vi "Get Param.vi"(3 "error in (no error)":errorcluster, 4 "param":dbl, 5 "paramID":i32) -> (0 "error out":errorcluster, 1 "param out":dbl, 2 "function return":i32)   [LabVIEW 2014, in "ThorZStepper.lvlib"]
doc: "long GetParam(const long paramID, double &param);"
uses:
  ThorZStepper.lvlib
  ThorZStepper.dll
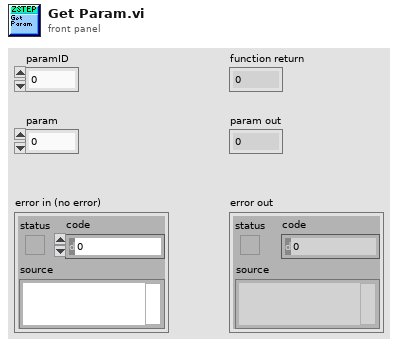
[diagram p1: front panel]
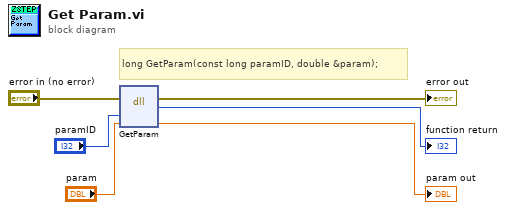
[diagram p0: block diagram]
diagram:
  # "long GetParam(const long paramID, double &param);"
  n1 = dll-call lib="C:/TIS_CalebVS2012/TIS_Development/Hardware/SDKs/MFC1_SDK/LabVIEW/inc/ThorZStepper.*" fn="GetParam"(error in="error in (no error)", "paramID"="paramID", "param"="param") -> (error out=→"error out":errorcluster, "return type"=→"function return":i32, "param"=→"param out":dbl)  [unwired: 3 in, 1 out]
